vi "PID Veering.vi"(6 "Deviation":dbl, 7 "Current Distance":dbl=15.0 format="%#_13g", 8 "error in (no error)":errorcluster, 11 "Refnum's":T1={"Gyro"="Gyro", "Mtr 1"="LeftMtr", "Mtr 2"="RightMtr"}) -> (0 "error out":errorcluster)   [LabVIEW 2016]
uses:
  <vilib>/addons/control/pid/pid.llb/PID (DBL).vi
  <vilib>/addons/control/pid/NI_PID_pid.lvlib
panel:
  out "Waveform Graph":dbl[](graph)
  in  "V-D":dbl format="%#_13g"
  in  "V-I":dbl format="%#_13g"
  in  "V-P":dbl=0.06 format="%#_13g"
  in  "D-D":dbl format="%#_13g"
  in  "D-I":dbl format="%#_13g"
  in  "D-P":dbl=0.0007 format="%#_13g"
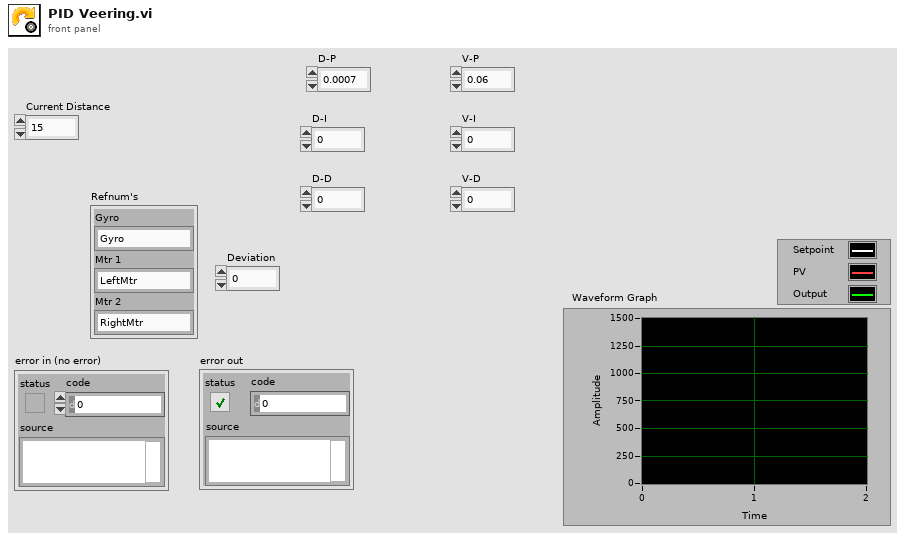
[diagram p1: front panel]
types:
  T1 = cluster{"Gyro":string, "Mtr 1":string, "Mtr 2":string}
  T2 = typedef "WPI_MotorControlDeviceRef.ctl" = cluster{"DeviceStatus":errorcluster, "Type":T3, "PWM":cluster{"PWM Channel":T4, "DeadBand":T5}, "CAN":cluster{"Device Number":u8, "SetOutput VI Ref":variant, "GetOutput VI Ref":variant, "Enable VI Ref":variant, "Disable VI Ref":variant, "Data":variant}, "Invert":bool}
  T3 = typedef "WPI_MotorControlType.ctl" = enum16{"PWM", "CAN"}
  T4 = typedef "FPGA_DIOPWMChannel.ctl" = enum8{"PWM 0", "PWM 1", "PWM 2", "PWM 3", "PWM 4", "PWM 5", "PWM 6", "PWM 7", "PWM 8", "PWM 9", "PWM MXP 0", "PWM MXP 1", "PWM MXP 2", "PWM MXP 3", "PWM MXP 4", "PWM MXP 5", "PWM MXP 6", "PWM MXP 7", "PWM MXP 8", "PWM MXP 9", "Invalid"}
  T5 = typedef "WPI_PWMDeadband.ctl" = cluster{"Name":string, "maxPositivePwm":i32, "minPositivePwm":i32, "centerPwm":i32, "maxNegativePwm":i32, "minNegativePwm":i32, "angularRange":u16}
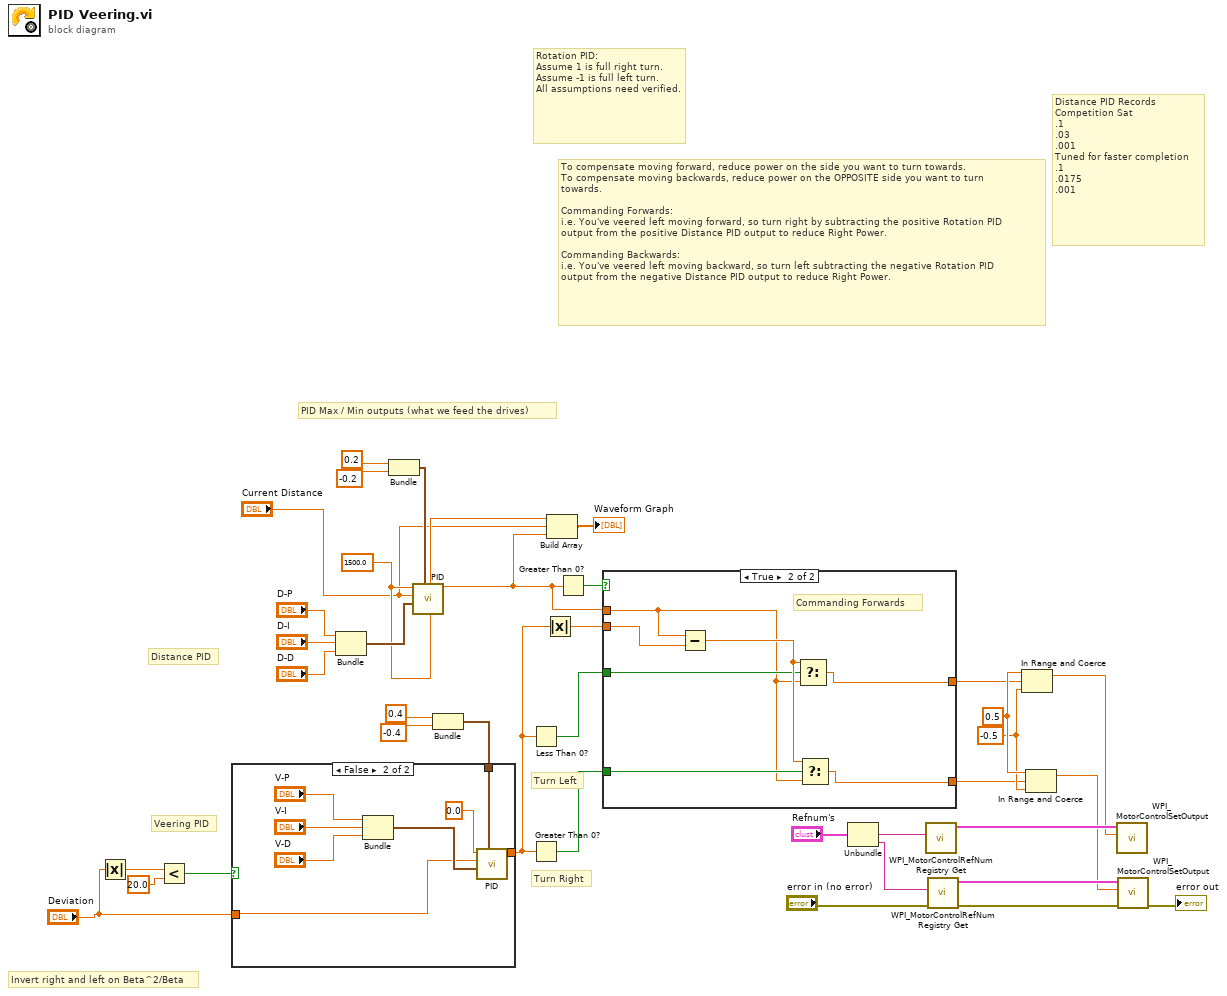
[diagram p0: block diagram]
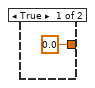
[diagram p2: hidden frame]
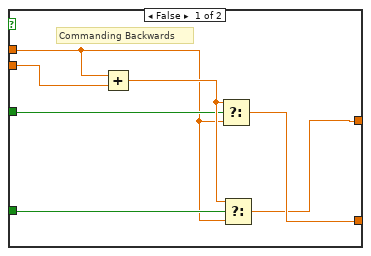
[diagram p3: hidden frame]
diagram:
  w11 = 1500.0 ("setpoint")
  w26 = -0.5
  w27 = 0.5
  # "Veering PID"
  # "Distance PID"
  # "Distance PID Records\nCompetition Sat\n.1\n.03\n.001\nTuned for faster completion\n.1\n.0175\n.001"
  # "Invert right and left on Beta^2/Beta"
  # "Turn Right"
  # "Turn Left"
  # "To compensate moving forward, reduce power on the side you want to turn towards.\nTo compensate moving backwards, reduce power on the OPPOSITE side you want to turn\ntowards.\n\nCommanding Forwards:\ni.e. You've veered left moving forward, so turn right by subtracting the positive Rotation PID\noutput from the positive Distance PID output to reduce Right Power.\n\nCommanding Backwards:\ni.e. You've veered left moving backward, so turn left subtracting the negative Rotation PID \noutput from the negative Distance PID output to reduce Right Power."
  # "PID Max / Min outputs (what we feed the drives)"
  # "Rotation PID:\nAssume 1 is full right turn.\nAssume -1 is full left turn.\nAll assumptions need verified."
  n1 = Absolute Value(x="Deviation") -> (abs(x)=w5:dbl)
  n2 = Less?(x=w5, y=20.0) -> (x < y?=w4:bool)
  n3 = Bundle("D-P"="D-P", "D-I"="D-I", "D-D"="D-D") -> (w30:cluster{"D-P":dbl, "D-I":dbl, "D-D":dbl})  [unwired: 1 in]
  n4 = Bundle(0.2, -0.2) -> (w29:cluster{dbl, dbl})  [unwired: 1 in]
  n5 = call-poly <vilib>:"PID.vi"("output range"=w29, "PID gains"=w30, "process variable"="Current Distance", "setpoint"=w11) -> ("output"=w9:dbl)  [unwired: 6 in, 1 out]
  n6 = Bundle(0.4, -0.4) -> (w1:cluster{dbl, dbl})  [unwired: 1 in]
  n7 = case shown="False" w4 {
    tunnel: w1 -> [_ w42]
    tunnel: [0.0 ("output") w41] -> w20
    tunnel: "Deviation" -> [_ w39]
    frame True {
    }
    frame False {
      n8 = Bundle("V-P"="V-P", "V-I"="V-I", "V-D"="V-D") -> (w43:cluster{"V-P":dbl, "V-I":dbl, "V-D":dbl})  [unwired: 1 in]
      n9 = call-poly <vilib>:"PID.vi"("output range"=w42, "PID gains"=w43, "process variable"=w39, "setpoint"=0.0) -> ("output"=w41:dbl)  [unwired: 6 in, 1 out]
    }
  }
  n10 = Less Than 0?(x=w20) -> (x < 0?=w22:bool)
  n11 = Greater Than 0?(x=w20) -> (x > 0?=w21:bool)
  n12 = Absolute Value(x=w20) -> (abs(x)=w25:dbl)
  n13 = Build Array(w11, "Current Distance", w9) -> (→"Waveform Graph":dbl[])
  n14 = Greater Than 0?(x=w9) -> (x > 0?=w28:bool)
  n15 = case shown="True" w28 {
    tunnel: w25 -> [w50 w60]
    tunnel: w9 -> [w47 w54]
    tunnel: [w49 w58] -> w24
    tunnel: [w48 w57] -> w23
    tunnel: w22 -> [w52 w56]
    tunnel: w21 -> [w51 w55]
    frame False {
      # "Commanding Backwards"
      n16 = Add(x=w47, y=w50) -> (x+y=w53:dbl)
      n17 = Select(t=w53, s=w52, f=w47) -> (s? t:f=w49:dbl)
      n18 = Select(t=w53, s=w51, f=w47) -> (s? t:f=w48:dbl)
    }
    frame True {
      # "Commanding Forwards"
      n19 = Subtract(x=w54, y=w60) -> (x-y=w59:dbl)
      n20 = Select(t=w59, s=w56, f=w54) -> (s? t:f=w57:dbl)
      n21 = Select(t=w59, s=w55, f=w54) -> (s? t:f=w58:dbl)
    }
  }
  n22 = Unbundle("Refnum's") -> ("Mtr 1"=w37:string, "Mtr 2"=w36:string)  [unwired: 1 out]
  n23 = call <vilib>:"WPI_MotorControlRefNum Registry Get.vi"("refnum name"=w37) -> ("MotorControlDevRef"=w17:T2)  [unwired: 9 in, 1 out]
  n24 = call <vilib>:"WPI_MotorControlRefNum Registry Get.vi"("error in (no error)"="error in (no error)", "refnum name"=w36) -> ("error out"=w12:errorcluster, "MotorControlDevRef"=w18:T2)  [unwired: 8 in]
  n25 = In Range and Coerce(upper limit=w27, x=w23, lower limit=w26) -> (coerced(x)=w16:dbl)  [unwired: 1 out]
  n26 = In Range and Coerce(upper limit=w27, x=w24, lower limit=w26) -> (coerced(x)=w15:dbl)  [unwired: 1 out]
  n27 = call <vilib>:"WPI_MotorControlSetOutput.vi"("Output"=w16, "MotorControlDevRef"=w17) -> ()  [unwired: 7 in, 3 out]
  n28 = call <vilib>:"WPI_MotorControlSetOutput.vi"("error in (no error)"=w12, "Output"=w15, "MotorControlDevRef"=w18) -> ("error out"=→"error out":errorcluster)  [unwired: 6 in, 2 out]
